vi "HPQ (SubVI).vi"(9 "B":dbl[](array[numeric]), 10 "A":dbl[](array[numeric]), 11 "Horizon":i32) -> (1 "H":T1, 2 "P":T1, 3 "Q":T1)   [LabVIEW 2016]
uses:
  <vilib>/Analysis/Matrix/Datatypes/RealMatrix.ctl
  <vilib>/Analysis/2dsp.llb/1D Convolution (DBL).vi
  <vilib>/Analysis/Matrix/Numeric/Conversions/Array To Matrix - RA.vi
  <vilib>/Analysis/Matrix/Numeric/Conversions/Array To Matrix - RA2.vi
  <vilib>/Analysis/7linalg.llb/Create Special Real Matrix.vi
  <vilib>/Analysis/baseanly.llb/Real Inverse Matrix.vi
  <vilib>/Analysis/Matrix/Numeric/Multiply/Multiply - RM,RM.vi
  <vilib>/Analysis/NI_AALPro.lvlib
  <vilib>/Analysis/Matrix/NI_Matrix.lvlib
  <vilib>/Analysis/NI_AALBase.lvlib
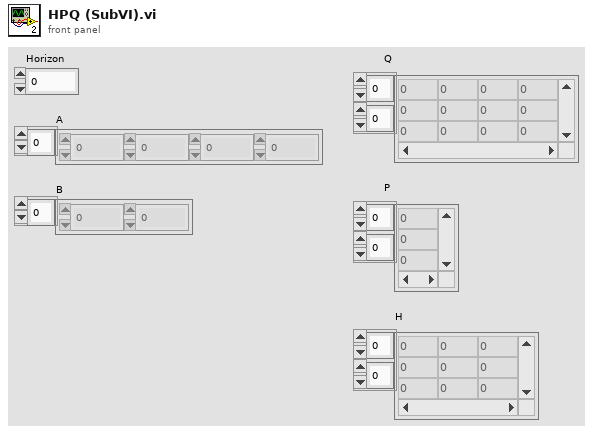
[diagram p1: front panel]
types:
  T1 = typedef "NI_Matrix.lvlib/RealMatrix.ctl" = dbl[][]
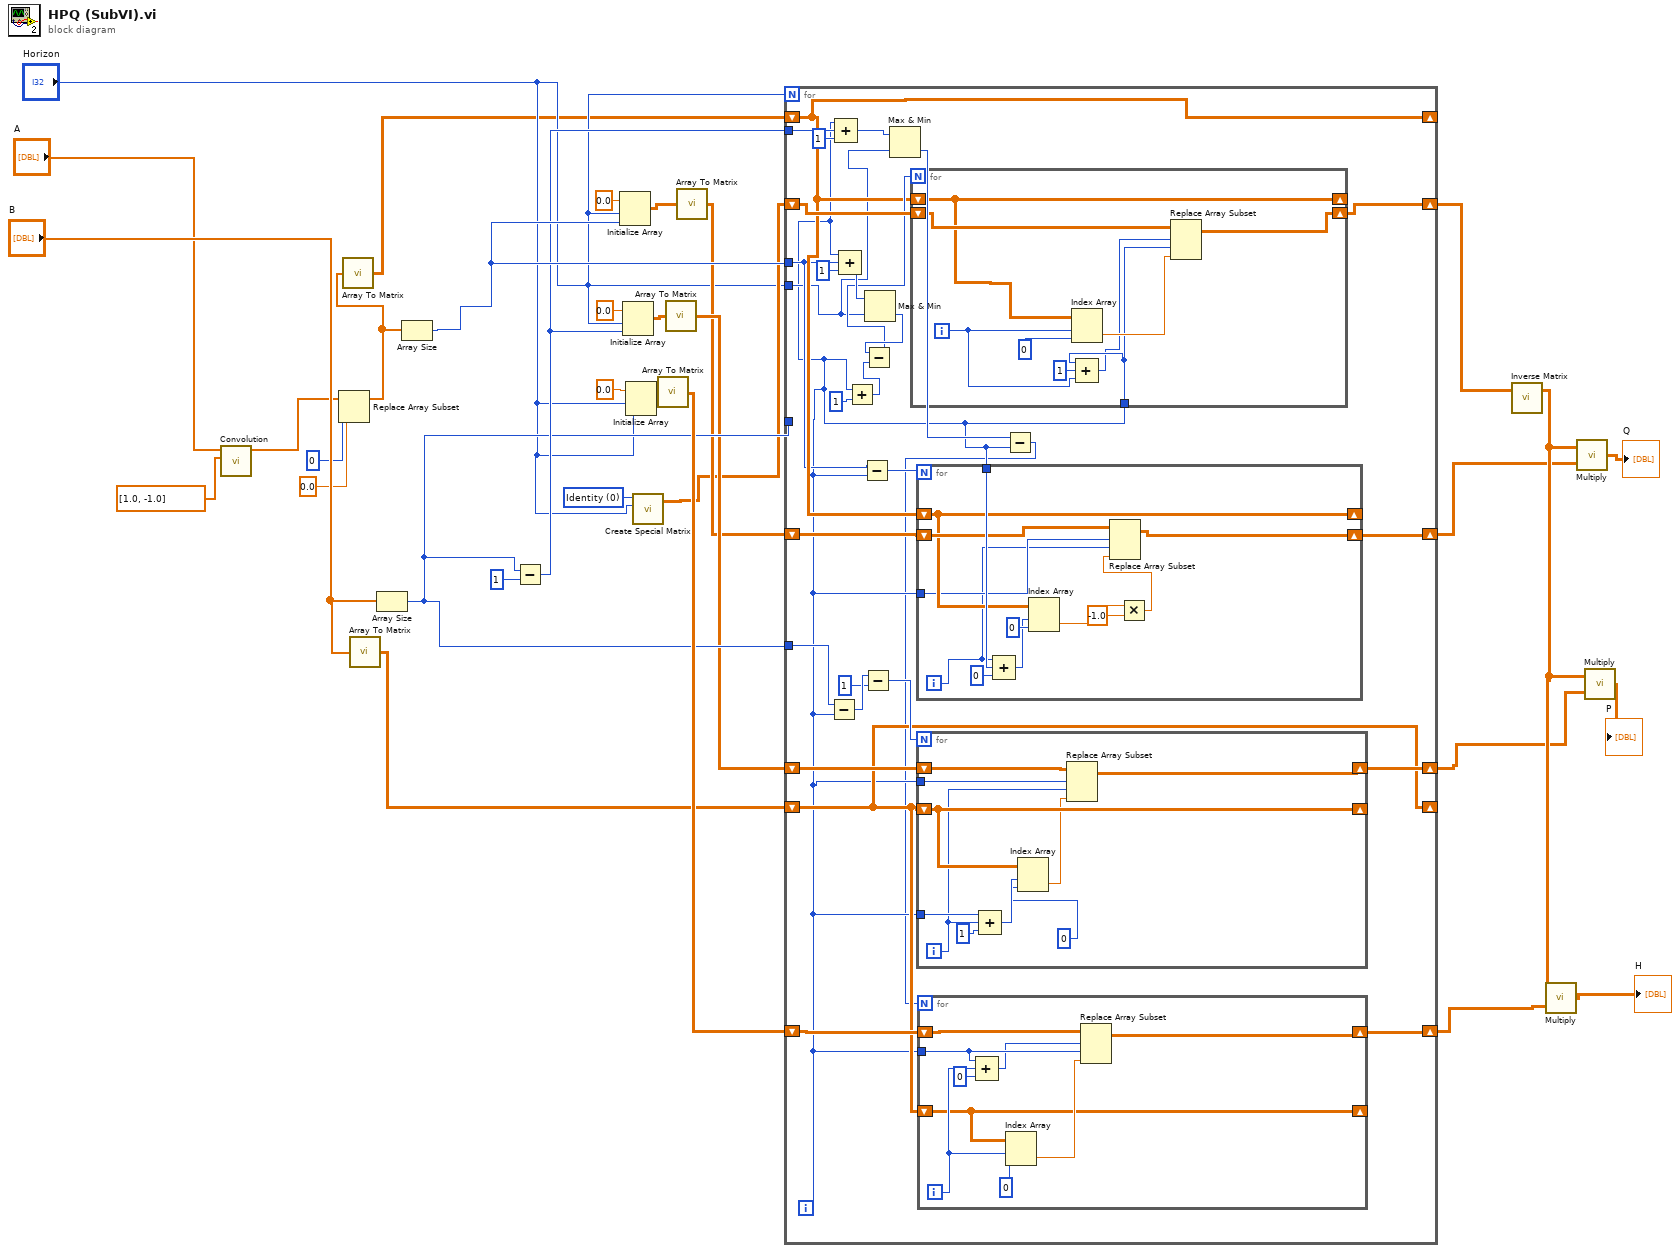
[diagram p0: block diagram]
diagram:
  w9 = 0 items=["Identity", "Diagonal", "Toeplitz", "Vandermonde", "Companion", "Hankel", "Hadamard", "Wilkinson", "Hilbert", "Inverse Hilbert", "Rosser", "Pascal"] ("matrix type")
  n1 = call-poly <vilib>:"Convolution.vi"("Y"=dbl[] [1.0, -1.0] ("A 2"), "X"="A") -> ("X * Y"=w3:dbl[])  [unwired: 8 in, 1 out]
  n2 = Replace Array Subset(array=w3, new element=0.0 ("new element/subarray"), index=0) -> (w13:dbl[])
  n3 = call-poly <vilib>:"Array To Matrix.vi"("Real 1D Array"=w13) -> ("Real Matrix (Column Vector)"=w14:T1)
  n4 = call-poly <vilib>:"Array To Matrix.vi"("Real 1D Array"="B") -> ("Real Matrix (Column Vector)"=w21:T1)
  n5 = Array Size(array="B") -> (size(s)=w22:i32)
  n6 = Array Size(array=w13) -> (size(s)=w33:i32)
  n7 = Subtract(x=w22, y=1) -> (x-y=w24:i32)
  n8 = Initialize Array(0.0 ("element"), "Horizon", w33) -> (w10:dbl[][])
  n9 = Initialize Array(0.0 ("element"), "Horizon", w24) -> (w11:dbl[][])
  n10 = Initialize Array(0.0 ("element"), "Horizon", "Horizon") -> (w12:dbl[][])
  n11 = call-poly <vilib>:"Create Special Matrix.vi"("matrix type"=w9, "matrix size"="Horizon") -> ("Special Matrix"=w17:T1)  [unwired: 3 in, 1 out]
  n12 = call-poly <vilib>:"Array To Matrix.vi"("Real 2D Array"=w12) -> ("Real Matrix"=w23:T1)
  n13 = call-poly <vilib>:"Array To Matrix.vi"("Real 2D Array"=w11) -> ("Real Matrix"=w19:T1)
  n14 = call-poly <vilib>:"Array To Matrix.vi"("Real 2D Array"=w10) -> ("Real Matrix"=w18:T1)
  n15 = for {
    N: "Horizon" -> [_]
    shift-right: [w61] -> w25
    shift-left: w17 -> [w62]
    shift-right: [w52] -> _
    shift-left: w14 -> [w52]
    tunnel: w22 -> [_]
    tunnel: w33 -> [w51]
    tunnel: "Horizon" -> [w40]
    shift-right: [w53] -> w26
    shift-left: w18 -> [w54]
    shift-right: [w48] -> w27
    shift-left: w19 -> [w49]
    shift-right: [w41] -> _
    shift-left: w21 -> [w41]
    tunnel: w22 -> [w47]
    shift-right: [w42] -> w29
    shift-left: w23 -> [w43]
    tunnel: w24 -> [w38]
    i -> [w35]
    n16 = Subtract(x=w47, y=w35) -> (x-y=w46:i32)
    n17 = Compound Arithmetic op=ADD(w35, w38, 1 ("value")) -> (w39:i32)
    n18 = Compound Arithmetic op=ADD(w35, w51, 1 ("value")) -> (w59:i32)
    n19 = Add(x=w35, y=1) -> (x+y=w56:i32)
    n20 = Subtract(x=w51, y=w35) -> (x-y=w50:i32)
    n21 = Subtract(x=w46, y=1) -> (x-y=w44:i32)
    n22 = Max & Min(x=w59, y=w40) -> (min(x,y)=w58:i32)  [unwired: 1 out]
    n23 = Subtract(x=w58, y=w56) -> (x-y=w55:i32)
    n24 = Max & Min(x=w39, y=w40) -> (min(x,y)=w36:i32)  [unwired: 1 out]
    n25 = for {
      N: w55 -> [_]
      shift-right: [w101] -> w61
      shift-left: w62 -> [w102]
      tunnel: w35 -> [w97]
      shift-right: [w100] -> _
      shift-left: w52 -> [w100]
      i -> [w95]
      n26 = Index Array(array=w100, index (row)=w95, index (col)=0 ("index (row)")) -> (element=w98:dbl)
      n27 = Compound Arithmetic op=ADD(w97, 1 ("value"), w95) -> (w94:i32)
      n28 = Replace Array Subset(array=w102, new element=w98, index (row)=w94, index (col)=w97) -> (w101:T1)
    }
    n29 = for {
      N: w50 -> [_]
      shift-right: [w88] -> w53
      shift-left: w54 -> [w89]
      shift-right: [w87] -> _
      shift-left: w52 -> [w87]
      tunnel: w35 -> [w92]
      tunnel: w35 -> [w86]
      i -> [w85]
      n30 = Compound Arithmetic op=ADD(w85, w92, 0 ("value")) -> (w90:i32)
      n31 = Index Array(array=w87, index (row)=w90, index (col)=0) -> (element=w83:dbl)
      n32 = Multiply(x=w83, y=-1.0) -> (x*y=w82:dbl)
      n33 = Replace Array Subset(array=w89, new element=w82, index (row)=w86, index (col)=w85) -> (w88:T1)
    }
    n34 = for {
      N: w44 -> [_]
      shift-right: [w79] -> w48
      shift-left: w49 -> [w80]
      shift-right: [w81] -> _
      shift-left: w41 -> [w81]
      tunnel: w35 -> [w77]
      tunnel: w35 -> [w75]
      i -> [w74]
      n35 = Compound Arithmetic op=ADD(w77, w74, 1 ("value")) -> (w73:i32)
      n36 = Index Array(array=w81, index (row)=w73, index (col)=0 ("index (row)")) -> (element=w76:dbl)
      n37 = Replace Array Subset(array=w80, new element=w76, index (row)=w75, index (col)=w74) -> (w79:T1)
    }
    n38 = Subtract(x=w36, y=w35) -> (x-y=w34:i32)
    n39 = for {
      N: w34 -> [_]
      shift-right: [w70] -> w42
      shift-left: w43 -> [w71]
      shift-right: [w63] -> _
      shift-left: w41 -> [w63]
      tunnel: w35 -> [w67]
      i -> [w66]
      n40 = Compound Arithmetic op=ADD(w67, w66, 0 ("value")) -> (w64:i32)
      n41 = Index Array(array=w63, index (row)=w66, index (col)=0) -> (element=w68:dbl)
      n42 = Replace Array Subset(array=w71, new element=w68, index (row)=w64, index (col)=w67) -> (w70:T1)
    }
  }
  n43 = call-poly <vilib>:"Inverse Matrix.vi"("Input Matrix"=w25) -> ("Inverse Matrix"=w30:T1)  [unwired: 1 in, 1 out]
  n44 = call-poly <vilib>:"Multiply.vi"("Real Matrix B"=w29, "Real Matrix A"=w30) -> ("A * B"=→"H":T1)
  n45 = call-poly <vilib>:"Multiply.vi"("Real Matrix B"=w26, "Real Matrix A"=w30) -> ("A * B"=→"Q":T1)
  n46 = call-poly <vilib>:"Multiply.vi"("Real Matrix B"=w27, "Real Matrix A"=w30) -> ("A * B"=→"P":T1)
